vi "Finish.vi"   [LabVIEW 2012]
doc: "This VI is called just before exiting. It is expected to close I/O refnum, save collected data, etc."
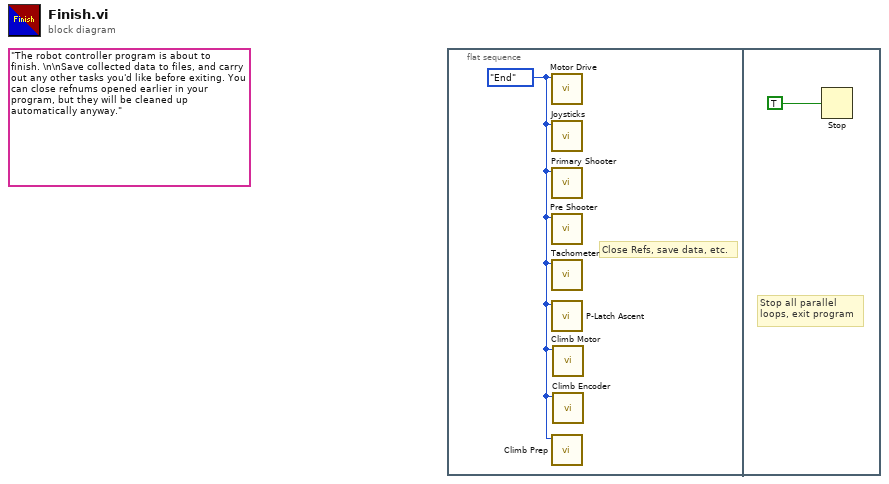
[diagram p0: block diagram]
diagram:
  (unwired) "The robot controller program is about to finish. \n\nSave collected data to files, and carry out any other tasks you'd like before exiting. You can close refnums opened earlier in your program, but they will be cleaned up automatically anyway."
  n1 = flat-sequence {
    frame #0 {
      w1 = enum16{"Start", "Run", "End"}."End" ("Enum")
      # "Close Refs, save data, etc."
      n2 = call "Motor Drive.vi"("Enum"=w1) -> ()  [unwired: 11 in]
      n3 = call "Joysticks.vi"("Enum"=w1) -> ()  [unwired: 9 in, 2 out]
      n4 = call "Primary Shooter.vi"("Enum"=w1) -> ()  [unwired: 11 in]
      n5 = call "Pre Shooter.vi"("Enum"=w1) -> ()  [unwired: 10 in]
      n6 = call "Tachometer.vi"("Enum"=w1) -> ()  [unwired: 10 in, 1 out]
      n7 = call "P-Latch Ascent.vi"("Enum"=w1) -> ()  [unwired: 10 in, 1 out]
      n8 = call "Climb Prep.vi"("Enum"=w1) -> ()  [unwired: 9 in, 2 out]
      n9 = call "Climb Motor.vi"("Enum"=w1) -> ()  [unwired: 11 in]
      n10 = call "Climb Encoder.vi"("Enum"=w1) -> ()  [unwired: 10 in, 1 out]
    }
    frame #1 {
      # "Stop all parallel\nloops, exit program"
      n11 = Stop(stop? (T)=TRUE ("Quit")) -> ()
    }
  }
